vi "AlarmQueryInstancesResponse_Parse.vi"(8 "error in (no error)":errorcluster, 11 "Message":T8) -> (0 "error out":errorcluster, 1 "Body":T1, 2 "Header":T7, 3 "AlarmQueryInstancesResponse":T6)   [LabVIEW 2017]
uses:
  <vilib>/addons/InsightCM/MessageBus/Base/controls/Message.ctl
  <vilib>/addons/InsightCM/MessageBus/Base/controls/MessageHeader.ctl
  <vilib>/addons/InsightCM/MessageBus/Base/controls/KeyValuePair.ctl
  <vilib>/addons/InsightCM/MessageBus/MessageLibrary/Alarm/controls/AlarmQueryInstancesResponse.ctl
  <vilib>/addons/InsightCM/MessageBus/MessageLibrary/Alarm/controls/AlarmQueryInstancesResponseBody.ctl
  <vilib>/addons/InsightCM/MessageBus/Base/controls/AlarmInstance.ctl
  <vilib>/addons/InsightCM/MessageBus/Base/controls/AlarmTransition.ctl
  <vilib>/addons/InsightCM/MessageBus/Base/controls/AlarmNote.ctl
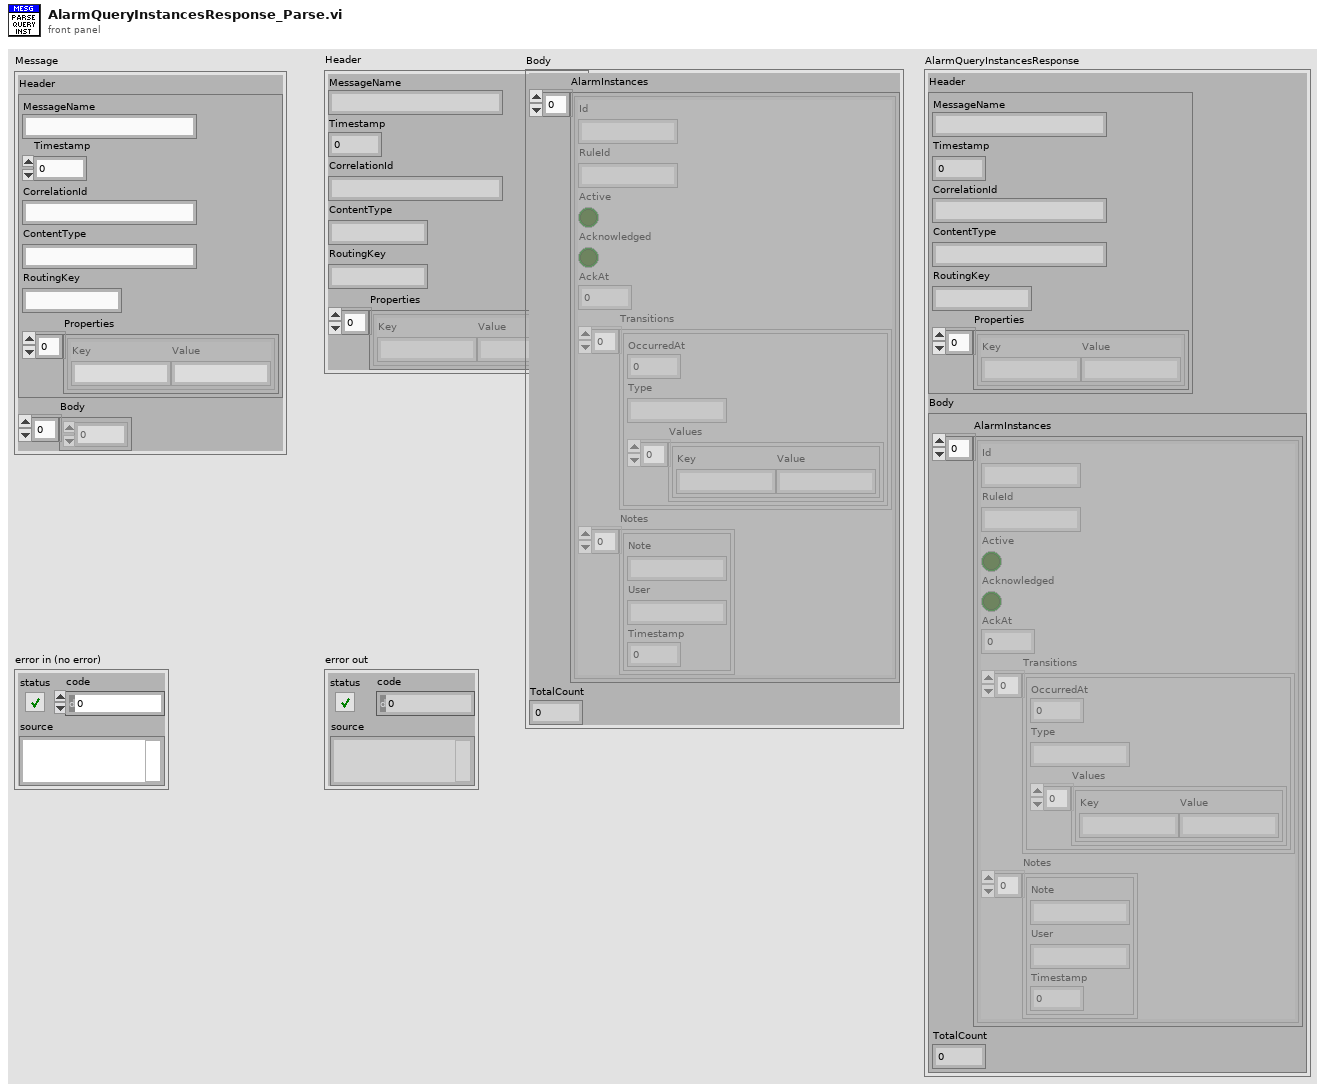
[diagram p1: front panel]
types:
  T1 = typedef "AlarmQueryInstancesResponseBody.ctl" = cluster{"AlarmInstances":T2[], "TotalCount":i32}
  T2 = typedef "AlarmInstance.ctl" = cluster{"Id":string, "RuleId":string, "Active":bool, "Acknowledged":bool, "AckAt":i64, "Transitions":T3[], "Notes":T5[]}
  T3 = typedef "AlarmTransition.ctl" = cluster{"OccurredAt":i64, "Type":string, "Values":T4[]}
  T4 = typedef "KeyValuePair.ctl" = cluster{"Key":string, "Value":string}
  T5 = typedef "AlarmNote.ctl" = cluster{"Note":string, "User":string, "Timestamp":i64}
  T6 = typedef "AlarmQueryInstancesResponse.ctl" = cluster{"Header":T7, "Body":T1}
  T7 = typedef "MessageHeader.ctl" = cluster{"MessageName":string, "Timestamp":i64, "CorrelationId":string, "ContentType":string, "RoutingKey":string, "Properties":T4[]}
  T8 = typedef "Message.ctl" = cluster{"Header":T7, "Body":u8[]}
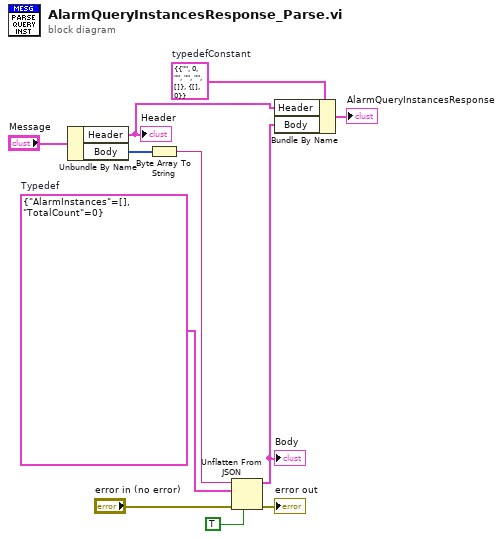
[diagram p0: block diagram]
diagram:
  w3 = T6 {"Header"={"MessageName"="", "Timestamp"=0, "CorrelationId"="", "ContentType"="", "RoutingKey"="", "Properties"=[]}, "Body"={"AlarmInstances"=[], "TotalCount"=0}}  # typedefConstant
  w7 = T1 {"AlarmInstances"=[], "TotalCount"=0}  # Typedef
  n1 = Unbundle By Name("Message") -> ("Header"=w9:T7, "Body"=w1:u8[])
  "Header" <- w9
  n2 = Byte Array To String(unsigned byte array=w1) -> (string=w6:string)
  n3 = Unflatten From JSON(JSON string=w6, type and defaults=w7, default null elements? (F)=TRUE, error in (no error)="error in (no error)") -> (value=w5:T1, error out=→"error out":errorcluster)  [unwired: 3 in]
  "Body" <- w5
  n4 = Bundle By Name(cluster=w3, "Header"=w9, "Body"=w5) -> (→"AlarmQueryInstancesResponse":T6)
